vi "Set DAQ V.vi"(8 "error in (no error)":errorcluster, 10 "Set Voltage":variant, 11 "VoltageUpdate in":refnum<class "VoltageUpdate.lvclass">) -> (0 "error out":errorcluster, 3 "VoltageUpdate out":refnum<class "VoltageUpdate.lvclass">)   [LabVIEW 2016, in "VoltageUpdate.lvclass"]
uses:
  VoltageUpdate.lvclass
  VoltageUpdate.lvclass/VoltageUpdate.ctl
  <vilib>/DAQmx/write.llb/DAQmx Write (Analog DBL 1Chan 1Samp).vi
  <vilib>/DAQmx/miscellaneous.llb/DAQmx Fill In Error Info.vi
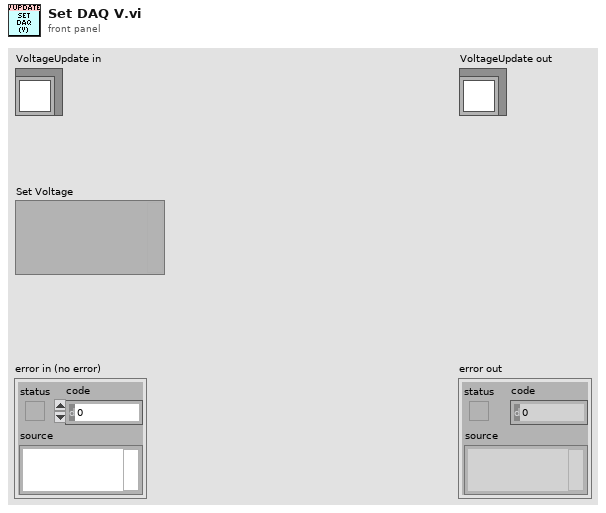
[diagram p1: front panel]
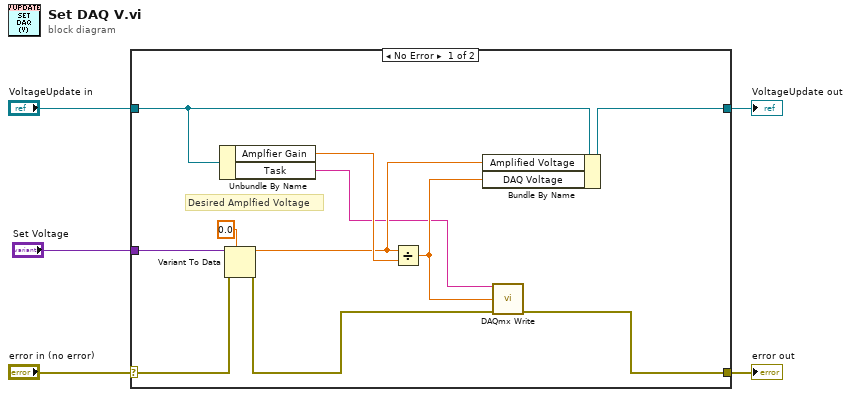
[diagram p0: block diagram]
diagram:
  n1 = case shown="No Error" "error in (no error)" {
    selector: "error in (no error)" -> [w15 w18]
    tunnel: [w8 w18] -> w4
    tunnel: [w11 w17] -> w2
    tunnel: "VoltageUpdate in" -> [w12 w17]
    tunnel: "Set Voltage" -> [w14 _]
    frame No Error {
      # "Desired Amplfied Voltage"
      n2 = Unbundle By Name(w12) -> ("Amplfier Gain"=w13:dbl, "Task"=w6:string)
      n3 = Variant To Data(error in=w15, type=0.0 ("data"), Variant=w14) -> (data=w10:dbl, error out=w9:errorcluster)
      n4 = Divide(x=w10, y=w13) -> (x/y=w7:dbl)
      n5 = Bundle By Name(cluster=w12, "Amplified Voltage"=w10, "DAQ Voltage"=w7) -> (w11:refnum<class "VoltageUpdate.lvclass">)
      n6 = call-poly <vilib>:"DAQmx Write.vi"("task/channels in"=w6, "data"=w7, "error in"=w9) -> ("error out"=w8:errorcluster)  [unwired: 10 in, 2 out]
    }
    frame Error {
    }
  }
  "error out" <- w4
  "VoltageUpdate out" <- w2
